vi "SVFA Power Spectral Density.vi"   [LabVIEW 2017]
doc: "Computes the power spectral density of <B>scaled signal [EU]</B> and returns the result in the selected units. Use the power spectral density to make repeatable measurements of the noise floor that are independent of the block size. Wire data to the <B>scaled signal [EU]</B> input to determine the polymorphic instance to use or manually select the instance."
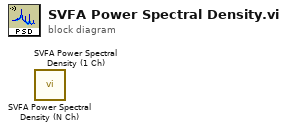
[diagram p0: block diagram]
diagram:
  n1 = call <vilib>:"SVFA Power Spectral Density (N Ch).vi"() -> ()  [unwired: 14 in, 6 out]
  n2 = call <vilib>:"SVFA Power Spectral Density (1 Ch).vi"() -> ()  [unwired: 14 in, 6 out]
